vi "Find_Invalid_Commands.vi"(1 "Alias Table":string[][](array[string]), 2 "Input Sequence":cluster{string, string[], dbl[], dbl}[](array[cluster])) -> (0 "Invalid Commands":string[](array[string]))   [LabVIEW 2011]
doc: "This VI examines the input growth sequence against the command alias table and outputs any commands for which an alias could not be found. These commands are invalid."
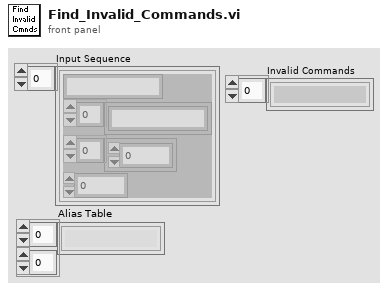
[diagram p1: front panel]
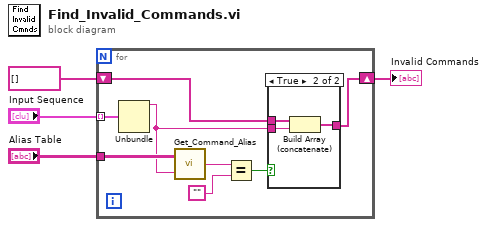
[diagram p0: block diagram]
diagram:
  n1 = for {
    tunnel: "Input Sequence" -> [w11] mode=indexing
    tunnel: "Alias Table" -> [w12]
    shift-right: [w8] -> w1
    shift-left: string[] [] -> [w7]
    n2 = Unbundle(w11) -> (w5:string)  [unwired: 3 out]
    n3 = call "Get_Command_Alias.vi"("Command"=w5, "Alias Table"=w12) -> ("Alias"=w9:string)
    n4 = Equal?(x=w9, y="") -> (x = y?=w6:bool)
    n5 = case shown="True" w6 {
      tunnel: w5 -> [_ w16]
      tunnel: [w13 w15] -> w8
      tunnel: w7 -> [w13 w14]
      frame False {
      }
      frame True {
        n6 = Build Array (concatenate)(w14, w16) -> (w15:string[])
      }
    }
  }
  "Invalid Commands" <- w1
